vi "Set Folder Hierarchy Writable.vi"(8 "error in (no error)":errorcluster, 11 "Folder Path (empty)":path) -> (0 "error out":errorcluster, 3 "dup Folder Path":path)   [LabVIEW 2011]
uses:
  OpenG/file/file.llb/File Exists - Scalar__ogtk.vi
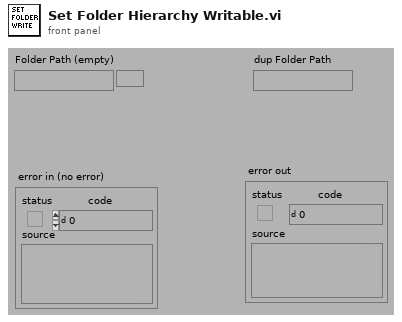
[diagram p1: front panel]
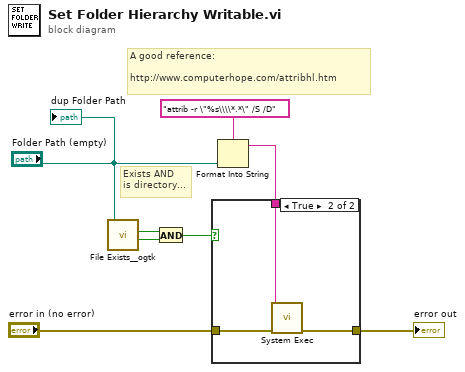
[diagram p0: block diagram]
diagram:
  # "Exists AND\nis directory..."
  # "A good reference:\n\nhttp://www.computerhope.com/attribhl.htm"
  n1 = call-poly "File Exists__ogtk.vi"("file path"="Folder Path (empty)") -> ("is directory"=w4:bool, "exists"=w3:bool)  [unwired: 6 in]
  n2 = And(x=w4, y=w3) -> (x .and. y?=w2:bool)
  n3 = Format Into String(format string="attrib -r \"%s\\\\*.*\" /S /D", "Folder Path (empty)") -> (resulting string=w8:string)  [unwired: 2 in, 1 out]
  n4 = case shown="True" w2 {
    tunnel: w8 -> [_ w12]
    tunnel: "error in (no error)" -> [w9 w11]
    tunnel: [w9 w10] -> w5
    frame False {
    }
    frame True {
      n5 = call <vilib>:"System Exec.vi"("error in (no error)"=w11, "command line"=w12) -> ("error out"=w10:errorcluster)  [unwired: 5 in, 4 out]
    }
  }
  "error out" <- w5
  "dup Folder Path" <- "Folder Path (empty)"
